vi "citTemplate.NextEvent.vi"(7 "instance":i32, 8 "error in":errorcluster, 10 "next event":variant, 11 "custom event":variant) -> (0 "error out":errorcluster)   [LabVIEW 2013]
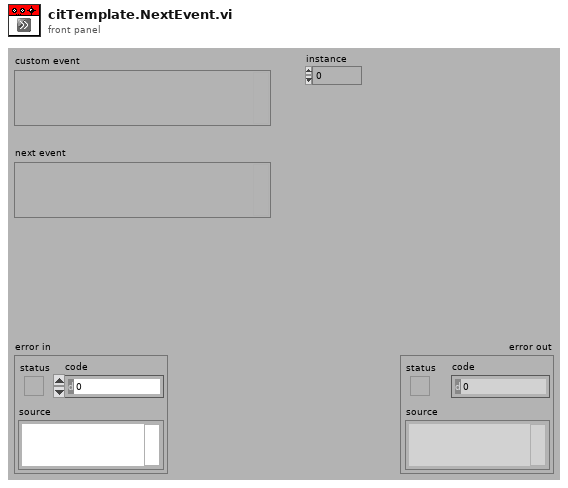
[diagram p1: front panel]
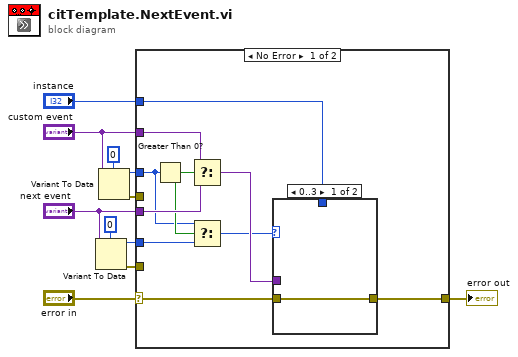
[diagram p0: block diagram]
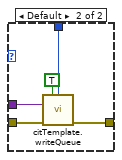
[diagram p2: hidden frame]
diagram:
  n1 = Variant To Data(type=u32 0 ("u32"), Variant="next event") -> (data=w7:u32, error out=w8:errorcluster)  [unwired: 1 in]
  n2 = Variant To Data(type=u32 0 ("u32"), Variant="custom event") -> (data=w4:u32, error out=w5:errorcluster)  [unwired: 1 in]
  n3 = case shown="No Error" "error in" {
    selector: "error in" -> [w18 w28]
    tunnel: [w21 w28] -> w10
    tunnel: "custom event" -> [w20 _]
    tunnel: "next event" -> [w19 _]
    tunnel: w8 -> [_ _]
    tunnel: w7 -> [w14 _]
    tunnel: w5 -> [_ _]
    tunnel: w4 -> [w15 _]
    tunnel: "instance" -> [w17 _]
    frame No Error {
      n4 = Greater Than 0?(x=w15) -> (x > 0?=w16:bool)
      n5 = Select(t=w20, s=w16, f=w19) -> (s? t:f=w13:variant)
      n6 = Select(t=w15, s=w16, f=w14) -> (s? t:f=w12:u32)
      n7 = case shown="0..3" w12 {
        tunnel: [w22 w27] -> w21
        tunnel: w18 -> [w22 w26]
        tunnel: w17 -> [_ w25]
        tunnel: w13 -> [_ w23]
        frame 0..3 {
        }
        frame Default {
          n8 = call "citTemplate.writeQueue.vi"("High priority (F)"=TRUE, "instance (0)"=w25, "event in (if not connected:all statemachine with data event)"=w23, "error in (no error)"=w26) -> ("error out"=w27:errorcluster)  [unwired: 1 in, 10 out]
        }
      }
    }
    frame Error {
    }
  }
  "error out" <- w10
